vi "Pcre2MatchDataCreateFromPattern8.vi"(8 "error in":errorcluster, 11 "pCode":u64 format="%.0x") -> (0 "error out":errorcluster, 2 "pMatchData":u64 format="%.0x", 3 "pCode":u64 format="%.0x")   [LabVIEW 2021, in "libpcre2-8.lvlib"]
uses:
  libpcre2-8.lvlib
  libpcre2-8-x32.dll
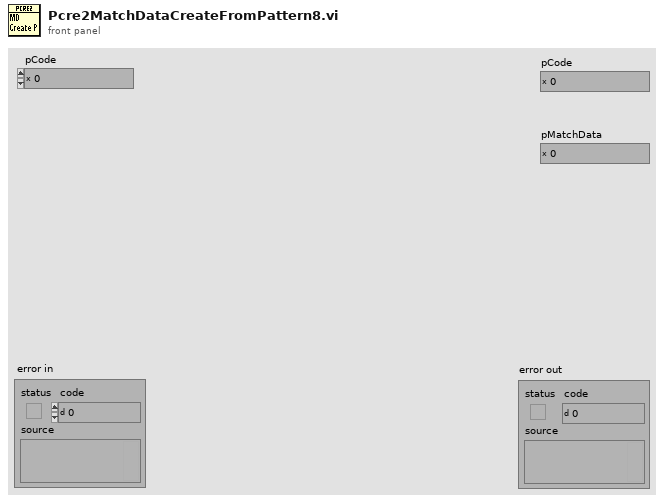
[diagram p1: front panel]
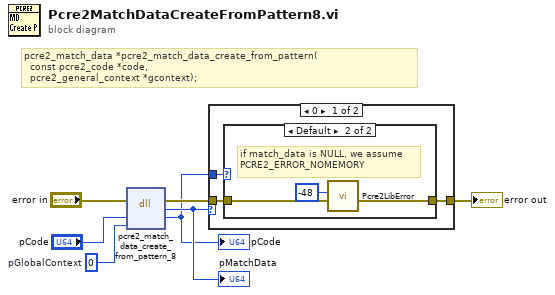
[diagram p0: block diagram]
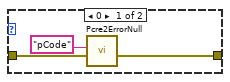
[diagram p2: hidden frame]
diagram:
  w7 = u64 0  # pGlobalContext
  # "pcre2_match_data *pcre2_match_data_create_from_pattern( \n  const pcre2_code *code, \n  pcre2_general_context *gcontext);"
  n1 = dll-call lib="libpcre2-8-x*.dll" fn="pcre2_match_data_create_from_pattern_8"(error in="error in", "code"="pCode", "gcontext"=w7) -> (error out=w2:errorcluster, "match_data"=w5:u64, "code"=w1:u64)  [unwired: 3 in, 1 out]
  "pCode" <- w1
  "pMatchData" <- w5
  n2 = case shown="0" w5 {
    tunnel: w2 -> [w9 w17]
    tunnel: [w10 w17] -> w6
    tunnel: w1 -> [w8 _]
    frame 0 {
      n3 = case shown="Default" w8 {
        tunnel: [w12 w16] -> w10
        tunnel: w9 -> [w13 w15]
        frame 0 {
          n4 = call "Pcre2ErrorNull.vi"("error in"=w13, "What"="pCode" ("message")) -> ("error out"=w12:errorcluster)  [unwired: 9 in]
        }
        frame Default {
          # "if match_data is NULL, we assume\nPCRE2_ERROR_NOMEMORY"
          n5 = call "Pcre2LibError.vi"("error in"=w15, "ErrorCode"=-48) -> ("error out"=w16:errorcluster)  [unwired: 9 in]
        }
      }
    }
    frame Default {
    }
  }
  "error out" <- w6
